vi "Forward Status to Parent.vi"(8 "error in (no error)":errorcluster, 10 "Module Status":T1, 11 "Module in":refnum<class "Module.lvclass">) -> (0 "error out":errorcluster, 3 "Module out":refnum<class "Module.lvclass">)   [LabVIEW 2020, in "Volatus.lvlib" / "Module.lvclass"]
uses:
  Module.lvclass
  Module Status Update.ctl
  MessageQ/MessageQ.lvclass
  State.ctl
  Module.lvclass/Module.ctl
  MessageQ/MessageQ.lvclass/MessageQ.ctl
  Volatus.lvlib
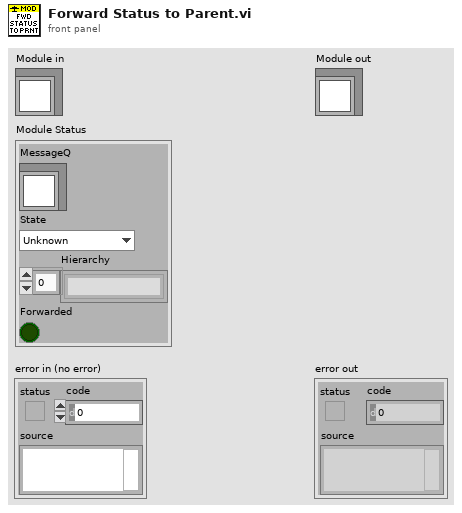
[diagram p1: front panel]
types:
  T1 = typedef "Volatus.lvlib/Module Status Update.ctl" = cluster{"MessageQ":refnum<class "MessageQ.lvclass">, "State":T2, "Hierarchy":string[], "Forwarded":bool}
  T2 = typedef "Volatus.lvlib/Module.lvclass/State.ctl" = enum16{"Unknown", "Launched", "Starting", "Running", "Stopping", "Stopped", "Error - Starting", "Error - Run", "Error - Stopping"}
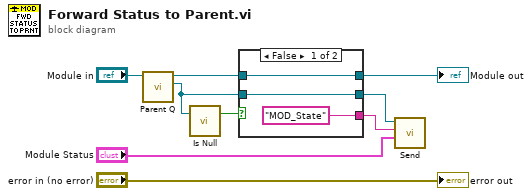
[diagram p0: block diagram]
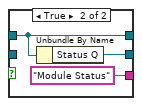
[diagram p2: hidden frame]
diagram:
  n1 = call "Parent Q.vi"("Module in"="Module in") -> ("Parent Q"=w6:refnum<class "MessageQ.lvclass">, "Module out"=w2:refnum<class "Module.lvclass">)  [unwired: 9 in]
  n2 = call "Is Null.vi"("MessageQ in"=w6) -> ("Null"=w7:bool)  [unwired: 2 in]
  n3 = case shown="False" w7 {
    tunnel: w6 -> [w11 _]
    tunnel: ["MOD_State" ("ID") "Module Status" ("ID")] -> w4
    tunnel: [w11 w13] -> w3
    tunnel: w2 -> [w10 w14]
    tunnel: [w10 w14] -> w1
    frame False {
    }
    frame True {
      n4 = Unbundle By Name(w14) -> ("Status Q"=w13:refnum<class "MessageQ.lvclass">)
    }
  }
  "Module out" <- w1
  n5 = call "Send.vi"("Data"="Module Status", "ID"=w4, "MessageQ in"=w3) -> ()  [unwired: 7 in, 2 out]
  "error out" <- "error in (no error)"
